vi "Connect to Error Handles.vi"(6 "Parent":refnum<vi>, 8 "error in":errorcluster, 10 "Timeout (ms)":u16, 11 "Process Names":string[](array[string])) -> (0 "error out":errorcluster, 3 "Error Handling Cluster":T1)   [LabVIEW 2015, in "Control Addon Engine.lvlib" / "Error Handling API.lvlib"]
uses:
  Error Handling API.lvlib
  Controls/Error Handling Cluster.ctl
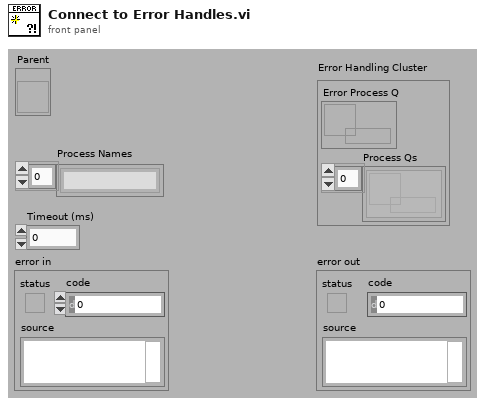
[diagram p1: front panel]
types:
  T1 = typedef "Control Addon Engine.lvlib/Error Handling API.lvlib/Error Handling Cluster.ctl" = cluster{"Error Process Q":refnum<queue>, "Process Qs":refnum<queue>[]}
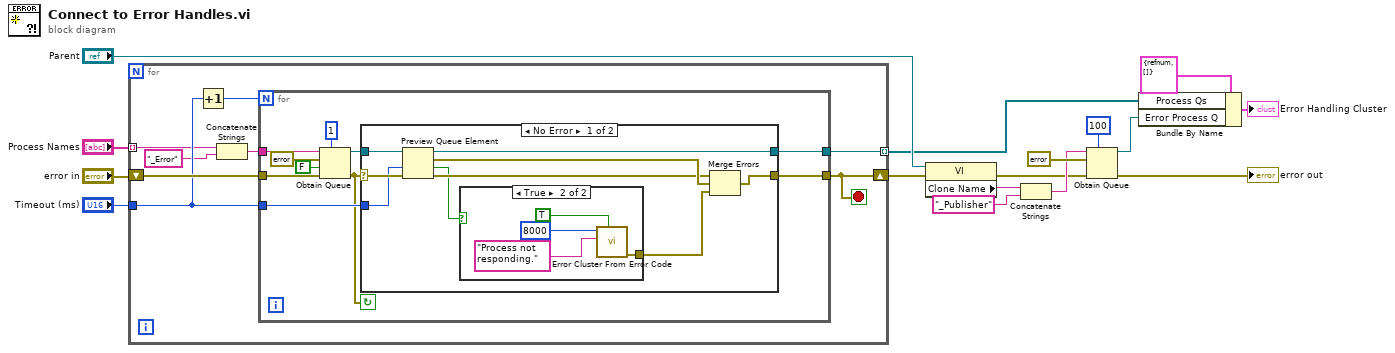
[diagram p0: block diagram]
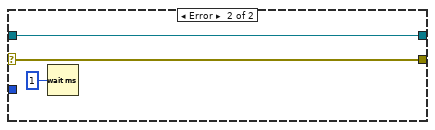
[diagram p3: hidden frame]
diagram:
  n1 = for {
    tunnel: "Process Names" -> [w20] mode=indexing
    shift-right: [w17] -> w11
    shift-left: "error in" -> [w24]
    tunnel: [w23] -> w2 mode=indexing
    tunnel: "Timeout (ms)" -> [w21]
    stop <- w17 stop-if-true
    n2 = Increment(x=w21) -> (x+1=w22:u16)
    n3 = Concatenate Strings(w20, "_Error" ("string")) -> (w18:string)
    n4 = for {
      N: w22 -> [_]
      tunnel: w18 -> [w34]
      tunnel: [w29] -> w23
      tunnel: w21 -> [w27]
      tunnel: w24 -> [w31]
      tunnel: [w26] -> w17
      stop <- w25 continue-if-true
      n5 = Obtain Queue(max queue size (-1, unlimited)=1, name (unnamed)=w34, element data type=errorcluster {"status"=FALSE, "code"=0, "source"=""} ("error out"), create if not found? (T)=FALSE, error in (no error)=w31) -> (queue out=w28:refnum<queue>, error out=w25:errorcluster)  [unwired: 1 out]
      n6 = case shown="No Error" w25 {
        selector: w25 -> [w41 w50]
        tunnel: [w37 w50] -> w26
        tunnel: [w42 w49] -> w29
        tunnel: w28 -> [w43 w49]
        tunnel: w27 -> [w40 _]
        frame No Error {
          n7 = Preview Queue Element(queue=w43, timeout in ms (-1)=w40, error in (no error)=w41) -> (queue out=w42:refnum<queue>, element=w39:errorcluster, timed out?=w35:bool, error out=w38:errorcluster)
          n8 = case shown="True" w35 {
            tunnel: [_ w47] -> w36
            frame False {
            }
            frame True {
              n9 = call <vilib>:"Error Cluster From Error Code.vi"("show call chain? (False)"=TRUE, "error message (\"\")"="Process not responding." ("source"), "error code (0)"=8000) -> ("error out"=w47:errorcluster)  [unwired: 6 in]
            }
          }
          n10 = Merge Errors(w38, w39, w36) -> (w37:errorcluster)
        }
        frame Error {
          n11 = Wait (ms)(milliseconds to wait=u32 1) -> ()  [unwired: 1 out]
        }
      }
    }
  }
  n12 = property class="VI"(reference="Parent", error in=w11) -> (error out=w10:errorcluster, "Clone Name"=w13:string)  [unwired: 1 out]
  n13 = Concatenate Strings(w13, "_Publisher" ("name (unnamed)")) -> (w12:string)
  n14 = Obtain Queue(max queue size (-1, unlimited)=100, name (unnamed)=w12, element data type=errorcluster {"status"=FALSE, "code"=0, "source"=""} ("element"), error in (no error)=w10) -> (queue out=w4:refnum<queue>, error out=→"error out":errorcluster)  [unwired: 1 in, 1 out]
  n15 = Bundle By Name(cluster=T1 {"Error Process Q"=refnum, "Process Qs"=[]} ("Error Handling Cluster"), "Process Qs"=w2, "Error Process Q"=w4) -> (→"Error Handling Cluster":T1)
